vi "Step Update Table 4.3 to 5.0.vi"(8 "error in (no error)":errorcluster, 11 "Connection Refnum":T1) -> (0 "error out":errorcluster, 3 "Connection Refnum":T1)   [LabVIEW 2011]
uses:
  Summitek EXT/ODBC/SQL Controls/Connection Refnum.ctl
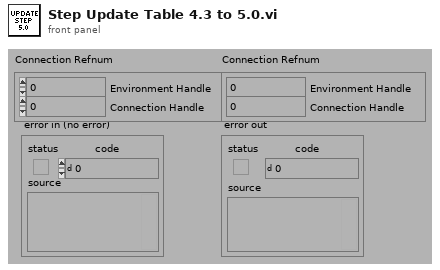
[diagram p1: front panel]
types:
  T1 = typedef "Connection Refnum.ctl" = cluster{"Environment Handle":i32, "Connection Handle":i32}
  T2 = typedef "Step Record.ctl" = cluster{"ixStep":i32, "sxSequenceId":string, "sxTestId":string, "iIndex":i32, "iRepeat":i32, "iQuickMode":i32, "sTag":string, "sDatasheetsCSV":string, "bConfiguration":string}
  T3 = typedef "Test Datasheets.ctl" = cluster{"Datasheet":string, "Print":bool}[]
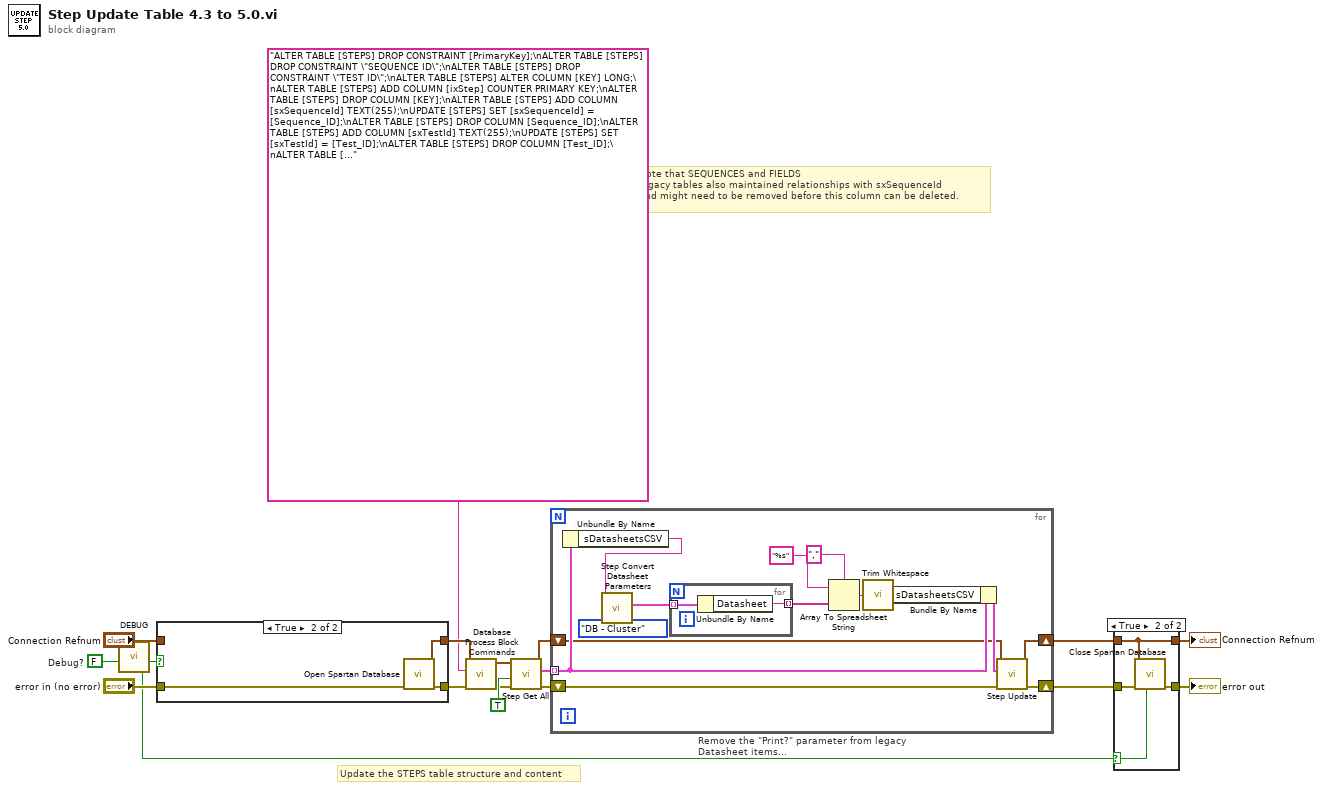
[diagram p0: block diagram]
diagram:
  w13 = FALSE  # Debug?
  # "Note that SEQUENCES and FIELDS\nlegacy tables also maintained relationships with sxSequenceId\nand might need to be removed before this column can be deleted."
  # "Update the STEPS table structure and content"
  n1 = call "DEBUG.vi"("Dev DEBUG? (f)"=w13) -> ("DEBUG?"=w12:bool)  [unwired: 1 in, 5 out]
  n2 = case shown="True" w12 {
    tunnel: "Connection Refnum" -> [w19 _]
    tunnel: "error in (no error)" -> [w18 w22]
    tunnel: [w18 w21] -> w11
    tunnel: [w19 w20] -> w3
    frame False {
    }
    frame True {
      n3 = call "Open Spartan Database.vi"("error in (no error)"=w22) -> ("error out"=w21:errorcluster, "Connection Refnum"=w20:T1)  [unwired: 2 in, 7 out]
    }
  }
  n4 = call "Database Process Block Commands.vi"("error in (no error)"=w11, "Database Commands (\"\")"="ALTER TABLE [STEPS] DROP CONSTRAINT [PrimaryKey];\nALTER TABLE [STEPS] DROP CONSTRAINT \"SEQUENCE ID\";\nALTER TABLE [STEPS] DROP CONSTRAINT \"TEST ID\";\nALTER TABLE [STEPS] ALTER COLUMN [KEY] LONG;\nALTER TABLE [STEPS] ADD COLUMN [ixStep] COUNTER PRIMARY KEY;\nALTER TABLE [STEPS] DROP COLUMN [KEY];\nALTER TABLE [STEPS] ADD COLUMN [sxSequenceId] TEXT(255);\nUPDATE [STEPS] SET [sxSequenceId] = [Sequence_ID];\nALTER TABLE [STEPS] DROP COLUMN [Sequence_ID];\nALTER TABLE [STEPS] ADD COLUMN [sxTestId] TEXT(255);\nUPDATE [STEPS] SET [sxTestId] = [Test_ID];\nALTER TABLE [STEPS] DROP COLUMN [Test_ID];\nALTER TABLE [STEPS] ADD COLUMN [iIndex] LONG;\nUPDATE [STEPS] SET [iIndex] = [Index];\nALTER TABLE [STEPS] DROP COLUMN [Index];\nALTER TABLE [STEPS] ADD COLUMN [iRepeat] LONG;\nUPDATE [STEPS] SET [iRepeat] = [Repeat_N];\nALTER TABLE [STEPS] DROP COLUMN [Repeat_N];\nALTER TABLE [STEPS] ADD COLUMN [iQuickMode] LONG;\nUPDATE [STEPS] SET [iQuickMode] = [QuickMode];\nALTER TABLE [STEPS] DROP COLUMN [QuickMode];\nALTER TABLE [STEPS] ADD COLUMN [sTag] TEXT(255);\nUPDATE [STEPS] SET [sTag] = [Tag];\nALTER TABLE [STEPS] DROP COLUMN [Tag];\nALTER TABLE [STEPS] ADD COLUMN [sDatasheetsCSV] MEMO;\nUPDATE [STEPS] SET [sDatasheetsCSV] = [Datasheets];\nALTER TABLE [STEPS] DROP COLUMN [Datasheets];\nALTER TABLE [STEPS] ADD COLUMN [bConfiguration] MEMO;\nUPDATE [STEPS] SET [bConfiguration] = [Configuration];\nALTER TABLE [STEPS] DROP COLUMN [Configuration];" ("User Query"), "Connection Refnum"=w3) -> ("error out"=w9:errorcluster, "Connection Refnum"=w2:T1)  [unwired: 7 out]
  n5 = call "Step Get All.vi"("error in (no error)"=w9, "All Steps? (f)"=TRUE, "Connection Refnum"=w2) -> ("error out"=w8:errorcluster, "Sequence Steps"=w7:T2[], "Connection Refnum"=w5:T1)  [unwired: 1 in, 5 out]
  n6 = for "Remove the \"Print?\" parameter from legacy Datasheet items..." {
    shift-right: [w35] -> w6
    shift-left: w8 -> [w36]
    tunnel: w7 -> [w34] mode=indexing
    shift-right: [w31] -> w4
    shift-left: w5 -> [w32]
    n7 = Unbundle By Name(w34) -> ("sDatasheetsCSV"=w30:string)
    n8 = call "Step Convert Datasheet Parameters.vi"("Conversion"=enum16{"DB - Cluster", "Cluster - DB"}."DB - Cluster", "Data String"=w30) -> ("Datasheets"=w28:T3)  [unwired: 1 in, 6 out]
    n9 = for {
      tunnel: w28 -> [w38] mode=indexing
      tunnel: [w37] -> w27 mode=indexing
      n10 = Unbundle By Name(w38) -> ("Datasheet"=w37:string)
    }
    n11 = Array To Spreadsheet String(delimiter (Tab)=",", array=w27, 3:"%s" ("format string")) -> (spreadsheet string=w24:string)
    n12 = call <vilib>:"Trim Whitespace.vi"("string"=w24) -> ("trimmed string"=w23:string)  [unwired: 1 in]
    n13 = Bundle By Name(cluster=w34, "sDatasheetsCSV"=w23) -> (w33:T2)
    n14 = call "Step Update.vi"("error in (no error)"=w36, "Step Record (empty)"=w33, "Connection Refnum"=w32) -> ("error out"=w35:errorcluster, "Connection Refnum"=w31:T1)  [unwired: 7 out]
  }
  n15 = case shown="True" w12 {
    selector: w12 -> [_ w42]
    tunnel: w6 -> [w40 w44]
    tunnel: w4 -> [w39 w41]
    tunnel: [w39 w41] -> w17
    tunnel: [w40 w43] -> w16
    frame False {
    }
    frame True {
      n16 = call "Close Spartan Database.vi"("Force Close? (f)"=w42, "error in (no error)"=w44, "Connection Refnum"=w41) -> ("error out"=w43:errorcluster)  [unwired: 2 in, 6 out]
    }
  }
  "error out" <- w16
  "Connection Refnum" <- w17
